vi "Connect.vi"(6 "Connect/Disconnect":bool, 8 "error in":errorcluster, 9 "Baud Rate":T1(ring), 10 "CAN Adapter Class Name":string, 11 "Interactor in":refnum<class "Interactor.lvclass">) -> (0 "error out":errorcluster, 3 "Interactor out":refnum<class "Interactor.lvclass">)   [LabVIEW 2024, in "Interactor.lvlib" / "Interactor.lvclass"]
uses:
  Interactor.lvclass
  Interactor.lvclass/Interactor.ctl
  Example/Home Messages/CAN Adapter Connected Msg/CAN Adapter Connected Msg.lvclass/CAN Adapter Connected Msg.ctl
  <vilib>/ActorFramework/Message Enqueuer/Message Enqueuer.lvclass/Message Enqueuer.ctl
  <vilib>/ActorFramework/Message Enqueuer/Enqueue.vi
  Example/Home Messages/CAN Adapter Connected Msg/CAN Adapter Connected Msg.lvclass
  <vilib>/Utility/LVClass/Get LV Class Name.vi
  <resource>/AFDebug/Generate Trace for Message.vi
  <vilib>/ActorFramework/Message Priority Queue/Priority Enqueue.vi
  CANopen Master/CANopen Master.lvclass
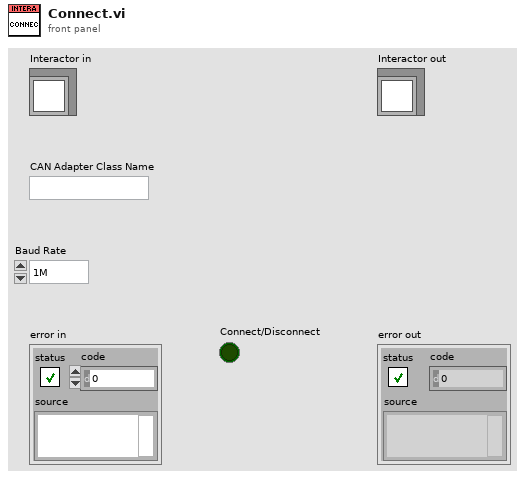
[diagram p1: front panel]
types:
  T1 = enum16{"1M", "800k", "500k", "250k", "125k", "50k", "25k", "10k"}
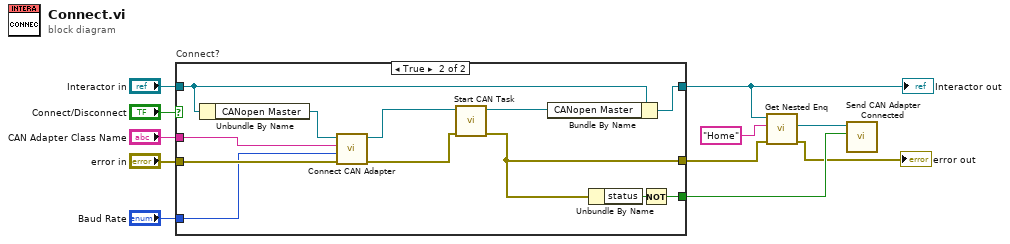
[diagram p0: block diagram]
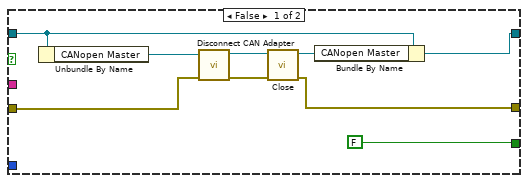
[diagram p2: hidden frame]
diagram:
  n1 = case "Connect?" shown="True" "Connect/Disconnect" {
    tunnel: "CAN Adapter Class Name" -> [_ w31]
    tunnel: "error in" -> [w19 w30]
    tunnel: "Interactor in" -> [w17 w25]
    tunnel: "Baud Rate" -> [_ w29]
    tunnel: [w14 w22] -> w4
    tunnel: [w13 w21] -> w1
    tunnel: [FALSE w27] -> w3
    frame False {
      n2 = Unbundle By Name(w17) -> ("CANopen Master"=w20:refnum<class "CANopen Master.lvclass">)
      n3 = call-dynamic "Disconnect CAN Adapter.vi"("error in"=w19, "CANopen Master in"=w20) -> ("error out"=w16:errorcluster, "CANopen Master out"=w15:refnum<class "CANopen Master.lvclass">)  [unwired: 8 in]
      n4 = call "Close.vi"("error in"=w16, "CANopen Master in"=w15) -> ("error out"=w14:errorcluster, "CANopen Master out"=w12:refnum<class "CANopen Master.lvclass">)  [unwired: 8 in]
      n5 = Bundle By Name(cluster=w17, "CANopen Master"=w12) -> (w13:refnum<class "Interactor.lvclass">)
    }
    frame True {
      n6 = Unbundle By Name(w25) -> ("CANopen Master"=w24:refnum<class "CANopen Master.lvclass">)
      n7 = call "Connect CAN Adapter.vi"("error in (no error)"=w30, "Baud Rate"=w29, "CAN Adapter Class Name"=w31, "CANopen Master in"=w24) -> ("error out"=w26:errorcluster, "CANopen Master out"=w32:refnum<class "CANopen Master.lvclass">)  [unwired: 6 in]
      n8 = call "Start CAN Task.vi"("error in"=w26, "CANopen Master in"=w32) -> ("error out"=w22:errorcluster, "CANopen Master out"=w23:refnum<class "CANopen Master.lvclass">)  [unwired: 8 in]
      n9 = Bundle By Name(cluster=w25, "CANopen Master"=w23) -> (w21:refnum<class "Interactor.lvclass">)
      n10 = Unbundle By Name(w22) -> ("status"=w28:bool)
      n11 = Not(x=w28) -> (.not. x?=w27:bool)
    }
  }
  "Interactor out" <- w1
  n12 = call "Get Nested Enq.vi"("error in"=w4, "Ident"="Home", "Interactor in"=w1) -> ("error out"=→"error out":errorcluster, "Enq"=w6:refnum<class "Message Enqueuer.lvclass">)  [unwired: 6 in, 1 out]
  n13 = call "Send CAN Adapter Connected.vi"("CAN Adapter Connected?"=w3, "Message Enqueuer"=w6) -> ()  [unwired: 8 in, 2 out]
